vi "Flight time.vi"() -> ()   [LabVIEW 2014]
doc: "Target VI used in conjunction with the asynchronous call examples."
panel:
  out "기록":string[](array[string])
  in  "닫기":bool
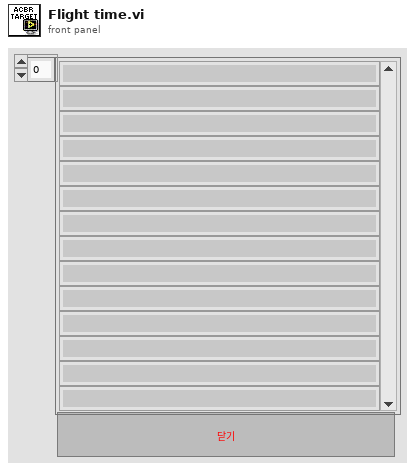
[diagram p1: front panel]
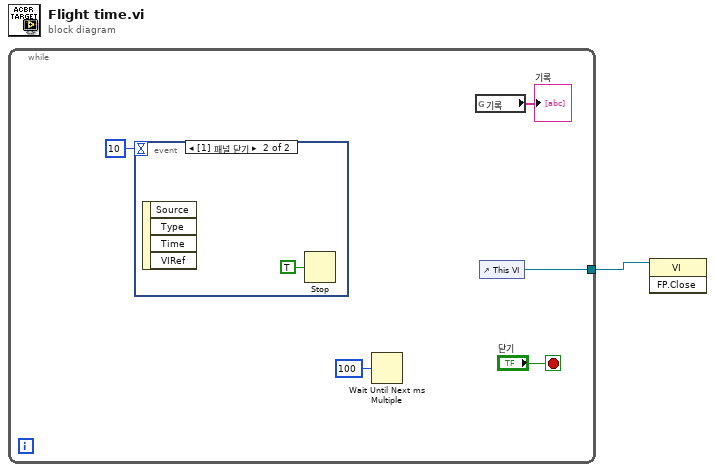
[diagram p0: block diagram]
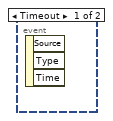
[diagram p2: hidden frame]
diagram:
  n1 = while {
    tunnel: [w5] -> w1
    stop <- "닫기" stop-if-true
    n2 = event shown="[1] 패널 닫기" {
      selector: _ -> [_ _]
      dyn-events: _ -> [_ _]
      timeout: 10 -> [_ _]
      event Timeout {
        n3 = event-data() -> ()  [unwired: 1 in, 3 out]
      }
      event Panel Close {
        n4 = event-data() -> ()  [unwired: 1 in, 4 out]
        n5 = Stop(stop? (T)=TRUE ("정지? (참)")) -> ()
      }
    }
    n6 = Wait Until Next ms Multiple(millisecond multiple=u32 100 ("ms 배수")) -> ()  [unwired: 1 out]
    n7 = global read "글로벌플라이트플랜.vi" "기록"() -> (→"기록":string[])
    n8 = control-ref of="This VI"() -> (w5:refnum<vi>)
  }
  n9 = invoke class="VI" method="FP.Close"(reference=w1) -> ()  [unwired: 2 in, 3 out]
